vi "CTRL Size Front Panel Object.vi"(4 "error in (no error)":errorcluster, 5 "Y":i32, 6 "x":i32, 7 "GObj Refnum":refnum<vi>) -> (0 "error out":errorcluster, 1 "new height":i32, 2 "new width":i32, 3 "GObj Refnum out":refnum<vi>)   [LabVIEW 2019]
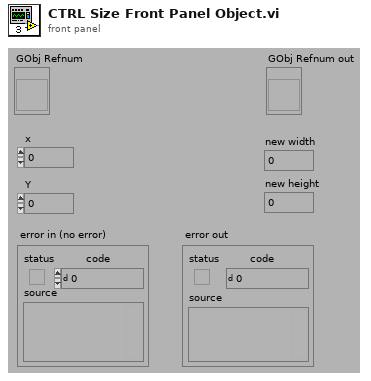
[diagram p1: front panel]
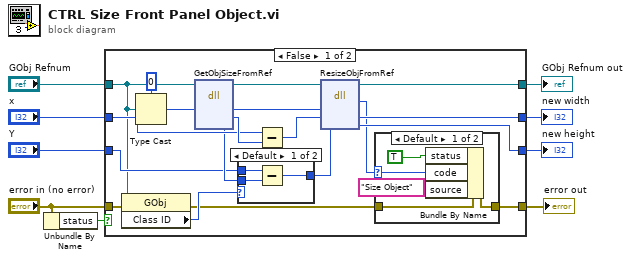
[diagram p0: block diagram]
diagram:
  n1 = Unbundle By Name("error in (no error)") -> ("status"=w1:bool)
  n2 = case shown="False" w1 {
    tunnel: "x" -> [w20 w38]
    tunnel: "Y" -> [w18 w37]
    tunnel: [w16 w38] -> w7
    tunnel: [w15 w37] -> w6
    tunnel: "GObj Refnum" -> [w10 w39]
    tunnel: "error in (no error)" -> [w13 w36]
    tunnel: [w11 w36] -> w4
    tunnel: [w10 w39] -> w3
    frame False {
      n3 = property class="GObj"(reference=w10, error in=w13) -> (error out=w12:errorcluster, "Class ID"=w23:u32)  [unwired: 1 out]
      n4 = Type Cast(type=0, x=w10) -> (*(type *) &x=w26:i32)
      n5 = dll-call lib="LabVIEW" fn="GetObjSizeFromRef"("objRef"=w26) -> ("objRef"=w24:i32, "width"=w22:i32, "height"=w19:i32)  [unwired: 6 in, 2 out]
      n6 = case shown="Default" w23 {
        tunnel: w19 -> [w35 _]
        tunnel: w18 -> [w34 _]
        tunnel: [w33 _] -> w17
        frame Default {
          n7 = Subtract(x=w34, y=w35) -> (x-y=w33:i32)
        }
        frame 32 {
        }
      }
      n8 = Subtract(x=w20, y=w22) -> (x-y=w21:i32)
      n9 = dll-call lib="LabVIEW" fn="ResizeObjFromRef"("ref"=w24, "deltaHoriz"=w21, "deltaVert"=w17) -> ("mgErr"=w14:i32, "deltaHoriz"=w16:i32, "deltaVert"=w15:i32)  [unwired: 4 in, 2 out]
      n10 = case shown="Default" w14 {
        selector: w14 -> [w29 _]
        tunnel: w12 -> [w31 w32]
        tunnel: [w30 w32] -> w11
        frame Default {
          n11 = Bundle By Name(cluster=w31, "status"=TRUE, "code"=w29, "source"="Size Object") -> (w30:errorcluster)
        }
        frame 0 {
        }
      }
    }
    frame True {
    }
  }
  "GObj Refnum out" <- w3
  "new width" <- w7
  "new height" <- w6
  "error out" <- w4
